vi "NI PXI-4072 DMM Main Page.vi"(8 "error in (no error)":errorcluster, 11 "Node Ptr":T4 format="%.0x") -> (0 "error out":errorcluster)   [LabVIEW 2015, in "NI PXI-4072 DMM Custom Device.lvlib"]
uses:
  NI PXI-4072 DMM Custom Device.lvlib
  <vilib>/NI Veristand/Custom Device API/Custom Device Item Ref.ctl
  4072_CD_DMM Function.ctl
  <vilib>/NI Veristand/Custom Device API/Custom Device Channel.ctl
  <vilib>/NI Veristand/Custom Device API/Custom Device Channel Type.ctl
  4072_Global.vi
  <vilib>/NI Veristand/Custom Device API/Get Item Property (String).vi
  <vilib>/NI Veristand/Custom Device API/Get Item Property (U16).vi
  <vilib>/NI Veristand/Custom Device API/Get Item Property (I32).vi
  <vilib>/NI Veristand/Custom Device API/Set Item Property (U16).vi
  <vilib>/NI Veristand/Custom Device API/Set Item Property (Double).vi
  <vilib>/NI Veristand/Custom Device API/Set Item Property (String).vi
  <vilib>/NI Veristand/Custom Device API/Custom Device API.lvlib
panel:
  in  "Resolution in Digits":T1(ring)=enum."5 1/2"
  in  "Voltage Range":enum16{".1", "1", "10", "100", "300"}(ring)
  in  "Capacitance Range":T2(ring)
  in  "Resistance Range":enum16{"100", "1K", "10K", "1M", "10M", "100M"}(ring)
  in  "Processor":i32=-2 min=-2 max=64 step=1
  in  "Decimation":u16=1
  in  "Measurement Type":T3
  in  "Name of Device in MAX":string
  in  "Header":cluster{"Section Name":string}={"Section Name"="PXI-4072  Settings"}
  in  "Description":string
  in  "Custom Device Name":string
  in  "Delete":bool
  # "(-2 is Automatic)"
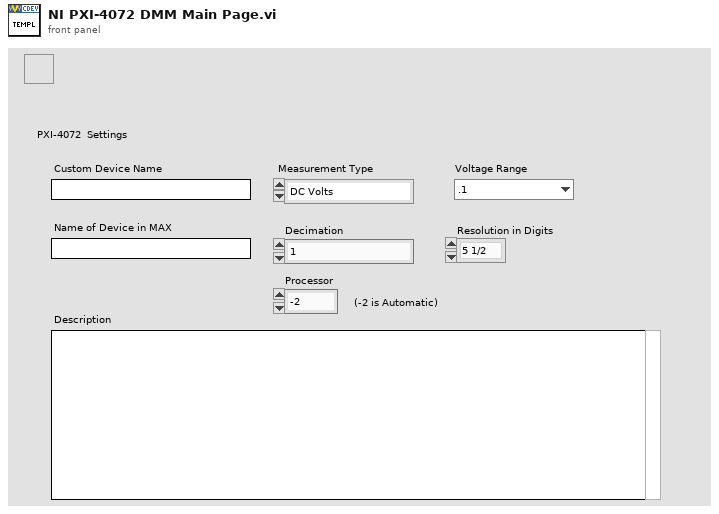
[diagram p1: front panel]
types:
  T1 = enum16{"3 1/2", "4 1/2", "5 1/2", "6 1/2", "7 1/7"}
  T2 = enum16{"300 pF", "1 nF", "10 nF", "100 nF", "1 uF", "10 uF", "100 uF", "1000 uF", "10000 uF"}
  T3 = typedef "NI PXI-4072 DMM Custom Device.lvlib/4072_CD_DMM Function.ctl" = enum16{"DC Volts", "2-wire Resistance", "4-wire Resistance", "Capacitance"}
  T4 = typedef "Custom Device API.lvlib/Custom Device Item Ref.ctl" = u64
  T5 = typedef "Custom Device API.lvlib/Custom Device Channel.ctl" = cluster{"Type":T6, "Units":string, "Default Value":dbl, "Faultable":bool, "Scalable":bool}
  T6 = typedef "Custom Device API.lvlib/Custom Device Channel Type.ctl" = enum16{"Input", "Output"}
  T7 = typedef "Custom Device API.lvlib/Custom Device Item Info.ctl" = cluster{"Name":string, "Is Channel":bool, "GUID":string, "Is Waveform":bool}
  T8 = typedef "Custom Device API.lvlib/Custom Device Commands.ctl" = enum16{"Default", "Item renamed", "Shutdown", "Dynamic button pressed"}
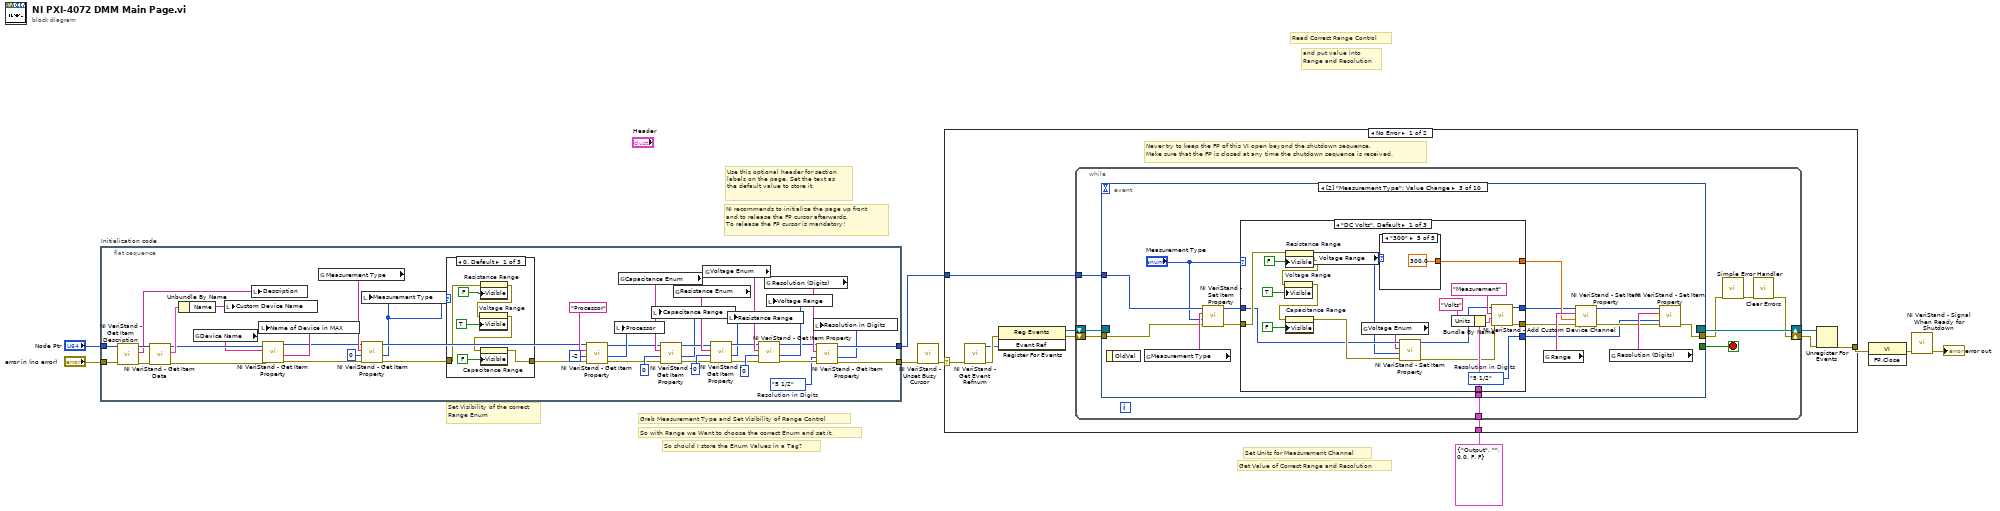
[diagram p0: block diagram]
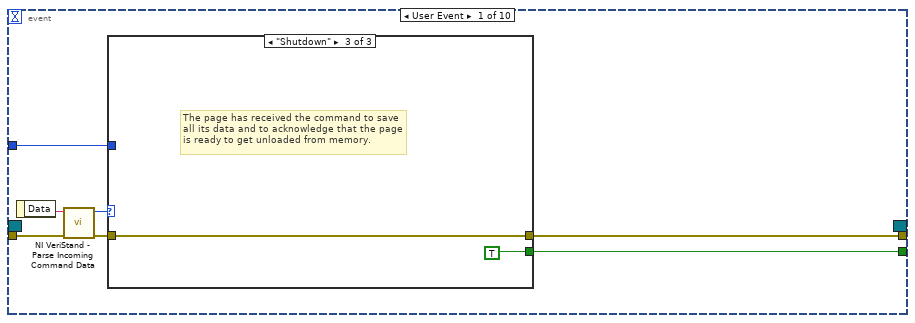
[diagram p2: hidden frame]
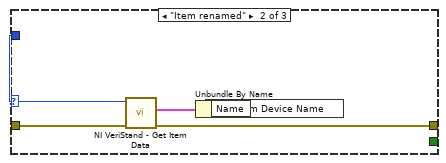
[diagram p4: hidden frame]
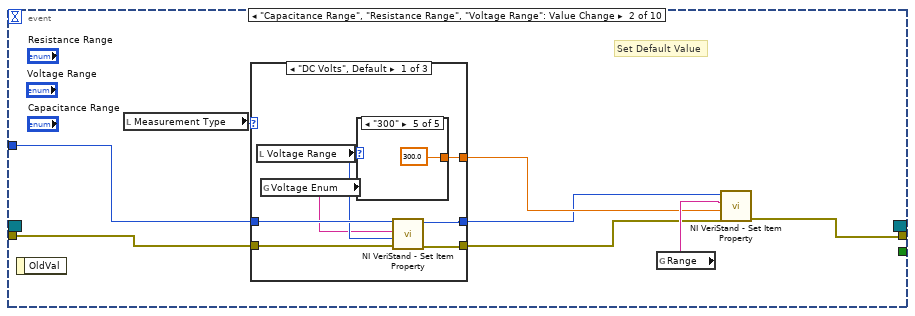
[diagram p5: hidden frame]
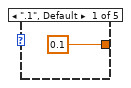
[diagram p6: hidden frame]
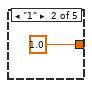
[diagram p7: hidden frame]
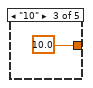
[diagram p8: hidden frame]
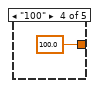
[diagram p9: hidden frame]
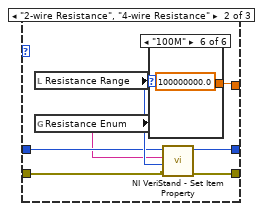
[diagram p10: hidden frame]
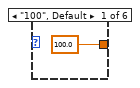
[diagram p11: hidden frame]
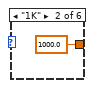
[diagram p12: hidden frame]
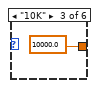
[diagram p13: hidden frame]
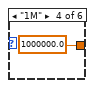
[diagram p14: hidden frame]
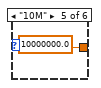
[diagram p15: hidden frame]
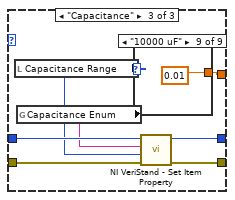
[diagram p16: hidden frame]
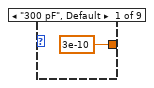
[diagram p17: hidden frame]
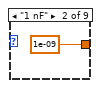
[diagram p18: hidden frame]
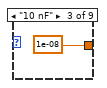
[diagram p19: hidden frame]
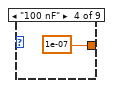
[diagram p20: hidden frame]
diagram:
  # "Set Units for Measurement Channel"
  # "Set Visibility of the correct\nRange Enum"
  # "Get Value of Correct Range and Resolution"
  # "So should I store the Enum Values in a Tag?"
  # "So with Range we Want to choose the correct Enum and set it."
  # "Grab Measurement Type and Set Visibility of Range Control"
  # "and put value into\nRange and Resolution"
  # "Read Correct Range Control"
  # "Use this optional header for section labels on the page. Set the text as the default value to store it."
  # "NI recommends to initialize the page up front\nand to release the FP cursor afterwards.\nTo release the FP cursor is mandatory!"
  n1 = flat-sequence "Initialization code" {
    tunnel: "error in (no error)" -> [w47]
    tunnel: "Node Ptr" -> [w48]
    tunnel: [w34] -> w5
    tunnel: [w35] -> w2
    frame #0 {
      w10 = T1."5 1/2"  # Resolution in Digits
      n2 = call <vilib>:"NI VeriStand - Get Item Description.vi"("error in (no error)"=w47, "Item Ref in"=w48) -> ("error out"=w51:errorcluster, "Description"=w52:string, "Item Ref out"=w53:T4)  [unwired: 7 out]
      n3 = call <vilib>:"NI VeriStand - Get Item Data.vi"("error in (no error)"=w51, "Item Ref in"=w53) -> ("error out"=w46:errorcluster, "Item Info"=w50:T7, "Item Ref out"=w45:T4)  [unwired: 7 out]
      n4 = Unbundle By Name(w50) -> ("Name"=w49:string)
      n5 = global read "4072_Global.vi" "Device Name"() -> (w44:string)
      n6 = local write "Custom Device Name"(w49) -> ()
      n7 = local write "Description"(w52) -> ()
      n8 = call-poly <vilib>:"NI VeriStand - Get Item Property.vi"("error in (no error)"=w46, "Property Name"=w44, "Item Ref in"=w45) -> ("error out"=w41:errorcluster, "Value"=w43:string, "Item Ref out"=w40:T4)  [unwired: 5 in, 1 out]
      n9 = local write "Name of Device in MAX"(w43) -> ()
      n10 = global read "4072_Global.vi" "Measurement Type"() -> (w42:string)
      n11 = call-poly <vilib>:"NI VeriStand - Get Item Property.vi"("error in (no error)"=w41, "Default Value"=u16 0, "Property Name"=w42, "Item Ref in"=w40) -> ("error out"=w13:errorcluster, "Value"=w14:u16, "Item Ref out"=w38:T4)  [unwired: 4 in, 1 out]
      n12 = local write "Measurement Type"(w14) -> ()
      n13 = case shown="0, Default" w14 {
        tunnel: w13 -> [w55 w61 w69]
        tunnel: [w54 w62 w68] -> w12
        frame 0, Default {
          n14 = property on="Resistance Range" class="Enum (strict)"(error in=w55, "Visible"=FALSE) -> (error out=w57:errorcluster)  [unwired: 1 in, 1 out]
          n15 = property on="Voltage Range" class="Enum (strict)"(error in=w57, "Visible"=TRUE) -> (error out=w56:errorcluster)  [unwired: 1 in, 1 out]
          n16 = property on="Capacitance Range" class="Enum (strict)"(error in=w56, "Visible"=FALSE) -> (error out=w54:errorcluster)  [unwired: 1 in, 1 out]
        }
        frame 1, 2 {
          n17 = property on="Resistance Range" class="Enum (strict)"(error in=w61, "Visible"=TRUE) -> (error out=w64:errorcluster)  [unwired: 1 in, 1 out]
          n18 = property on="Voltage Range" class="Enum (strict)"(error in=w64, "Visible"=FALSE) -> (error out=w63:errorcluster)  [unwired: 1 in, 1 out]
          n19 = property on="Capacitance Range" class="Enum (strict)"(error in=w63, "Visible"=FALSE) -> (error out=w62:errorcluster)  [unwired: 1 in, 1 out]
        }
        frame 3 {
          n20 = property on="Resistance Range" class="Enum (strict)"(error in=w69, "Visible"=FALSE) -> (error out=w71:errorcluster)  [unwired: 1 in, 1 out]
          n21 = property on="Voltage Range" class="Enum (strict)"(error in=w71, "Visible"=FALSE) -> (error out=w70:errorcluster)  [unwired: 1 in, 1 out]
          n22 = property on="Capacitance Range" class="Enum (strict)"(error in=w70, "Visible"=TRUE) -> (error out=w68:errorcluster)  [unwired: 1 in, 1 out]
        }
      }
      n23 = call-poly <vilib>:"NI VeriStand - Get Item Property.vi"("error in (no error)"=w12, "Default Value"=-2, "Property Name"="Processor", "Item Ref in"=w38) -> ("error out"=w24:errorcluster, "Value"=w37:i32, "Item Ref out"=w27:T4)  [unwired: 4 in, 1 out]
      n24 = local write "Processor"(w37) -> ()
      n25 = global read "4072_Global.vi" "Capacitance Enum"() -> (w33:string)
      n26 = call-poly <vilib>:"NI VeriStand - Get Item Property.vi"("error in (no error)"=w24, "Default Value"=0, "Property Name"=w33, "Item Ref in"=w27) -> ("error out"=w23:errorcluster, "Value"=w19:u16, "Item Ref out"=w26:T4)  [unwired: 4 in, 1 out]
      n27 = local write "Capacitance Range"(w19) -> ()
      n28 = global read "4072_Global.vi" "Resistance Enum"() -> (w32:string)
      n29 = global read "4072_Global.vi" "Voltage Enum"() -> (w31:string)
      n30 = call-poly <vilib>:"NI VeriStand - Get Item Property.vi"("error in (no error)"=w23, "Default Value"=0, "Property Name"=w32, "Item Ref in"=w26) -> ("error out"=w22:errorcluster, "Value"=w18:u16, "Item Ref out"=w25:T4)  [unwired: 4 in, 1 out]
      n31 = local write "Resistance Range"(w18) -> ()
      n32 = call-poly <vilib>:"NI VeriStand - Get Item Property.vi"("error in (no error)"=w22, "Default Value"=0, "Property Name"=w31, "Item Ref in"=w25) -> ("error out"=w21:errorcluster, "Value"=w20:u16, "Item Ref out"=w17:T4)  [unwired: 4 in, 1 out]
      n33 = global read "4072_Global.vi" "Resolution (Digits)"() -> (w36:string)
      n34 = local write "Voltage Range"(w20) -> ()
      n35 = call-poly <vilib>:"NI VeriStand - Get Item Property.vi"("error in (no error)"=w21, "Default Value"=w10, "Property Name"=w36, "Item Ref in"=w17) -> ("error out"=w34:errorcluster, "Value"=w11:u16, "Item Ref out"=w35:T4)  [unwired: 4 in, 1 out]
      n36 = local write "Resolution in Digits"(w11) -> ()
    }
  }
  n37 = call <vilib>:"NI VeriStand - Unset Busy Cursor.vi"("error in (no error)"=w5) -> ("error out"=w4:errorcluster)  [unwired: 10 out]
  n38 = case shown="No Error" w4 {
    selector: w4 -> [w76 w286]
    tunnel: [w81 w284] -> w9
    tunnel: w2 -> [w77 _]
    tunnel: T5 {"Type"=enum."Output", "Units"="", "Default Value"=0.0, "Faultable"=FALSE, "Scalable"=FALSE} ("Channel") -> [w75 _]
    frame No Error {
      # "Never try to keep the FP of this VI open beyond the shutdown sequence.\nMake sure that the FP is closed at any time the shutdown sequence is received."
      n39 = call <vilib>:"NI VeriStand - Get Event Refnum.vi"("error in (no error)"=w76) -> ("error out"=w84:errorcluster, "Event Ref"=w80:refnum<user-event>)  [unwired: 9 out]
      n40 = register-events(error in=w84, w80) -> (reference out=w78:refnum<event-registration>, error out=w79:errorcluster)  [unwired: 1 in]
      n41 = while {
        tunnel: w77 -> [w89]
        shift-right: [w86] -> w82
        shift-left: w79 -> [w92]
        shift-right: [w93] -> w83
        shift-left: w78 -> [w91]
        tunnel: w75 -> [w85]
        stop <- w90 stop-if-true
        n42 = event shown="[2] \"Measurement Type\": Value Change" {
          selector: w91 -> [_ _ _ _ _ _ _ _ _ _]
          dyn-events: [_ _ _ _ _ _ _ _ _ _] -> w93
          timeout: _ -> [_ _ _ _ _ _ _ _ _ _]
          tunnel: w92 -> [w100 w111 w170 w256 w260 w265 w272 w276 w279 w283]
          tunnel: [w96 _ _ _ _ _ _ _ _ _] -> w90
          tunnel: [w95 w114 w164 w255 w259 w264 w268 w275 w278 w282] -> w88
          tunnel: w89 -> [w94 w112 w171 w257 w262 w266 w271 w274 w280 w281]
          tunnel: w85 -> [_ _ w158 _ _ _ _ _ _ _]
          event User Event {
            n43 = event-data() -> ("Data"=w99:string)  [unwired: 1 out]
            n44 = call <vilib>:"NI VeriStand - Parse Incoming Command Data.vi"("error in (no error)"=w100, "Incoming data"=w99) -> ("error out"=w98:errorcluster, "Action"=w97:T8)  [unwired: 8 out]
            n45 = case shown="\"Shutdown\"" w97 {
              tunnel: w98 -> [w101 w106 w107]
              tunnel: [_ _ TRUE] -> w96
              tunnel: [w101 w103 w107] -> w95
              tunnel: w94 -> [_ w105 _]
              frame "Default", Default {
              }
              frame "Item renamed" {
                n46 = call <vilib>:"NI VeriStand - Get Item Data.vi"("error in (no error)"=w106, "Item Ref in"=w105) -> ("error out"=w103:errorcluster, "Item Info"=w104:T7)  [unwired: 8 out]
                n47 = Unbundle By Name(w104) -> ("Name"=w102:string)
                n48 = local write "Custom Device Name"(w102) -> ()
              }
              frame "Shutdown" {
                # "The page has received the command to save all its data and to acknowledge that the page is ready to get unloaded from memory."
              }
            }
          }
          event "Capacitance Range", "Resistance Range", "Voltage Range": Value Change {
            # "Set Default Value"
            n49 = event-data() -> ()  [unwired: 2 out]
            n50 = local read "Measurement Type"() -> (w116:T3)
            n51 = case shown="\"DC Volts\", Default" w116 {
              tunnel: [w123 w135 w148] -> w113
              tunnel: w112 -> [w119 w133 w147]
              tunnel: w111 -> [w120 w130 w146]
              tunnel: [w121 w131 w145] -> w110
              tunnel: [w122 w132 w144] -> w109
              frame "DC Volts", Default {
                n52 = local read "Voltage Range"() -> (w118:enum16{".1", "1", "10", "100", "300"})
                n53 = global read "4072_Global.vi" "Voltage Enum"() -> (w117:string)
                n54 = case shown="\"300\"" w118 {
                  tunnel: [0.1 1.0 10.0 100.0 300.0] -> w123
                  frame ".1", Default {
                  }
                  frame "1" {
                  }
                  frame "10" {
                  }
                  frame "100" {
                  }
                  frame "300" {
                  }
                }
                n55 = call-poly <vilib>:"NI VeriStand - Set Item Property.vi"("error in (no error)"=w120, "Value"=w118, "Property Name"=w117, "Item Ref in"=w119) -> ("error out"=w121:errorcluster, "Item Ref out"=w122:T4)  [unwired: 5 in, 1 out]
              }
              frame "2-wire Resistance", "4-wire Resistance" {
                n56 = local read "Resistance Range"() -> (w134:enum16{"100", "1K", "10K", "1M", "10M", "100M"})
                n57 = global read "4072_Global.vi" "Resistance Enum"() -> (w129:string)
                n58 = case shown="\"100M\"" w134 {
                  tunnel: [100.0 1000.0 10000.0 1000000.0 10000000.0 100000000.0] -> w135
                  frame "100", Default {
                  }
                  frame "1K" {
                  }
                  frame "10K" {
                  }
                  frame "1M" {
                  }
                  frame "10M" {
                  }
                  frame "100M" {
                  }
                }
                n59 = call-poly <vilib>:"NI VeriStand - Set Item Property.vi"("error in (no error)"=w130, "Value"=w134, "Property Name"=w129, "Item Ref in"=w133) -> ("error out"=w131:errorcluster, "Item Ref out"=w132:T4)  [unwired: 5 in, 1 out]
              }
              frame "Capacitance" {
                n60 = local read "Capacitance Range"() -> (w142:T2)
                n61 = global read "4072_Global.vi" "Capacitance Enum"() -> (w143:string)
                n62 = case shown="\"10000 uF\"" w142 {
                  tunnel: [3e-10 1e-09 1e-08 1e-07 1e-06 1e-05 0.0001 0.001 0.01] -> w148
                  frame "300 pF", Default {
                  }
                  frame "1 nF" {
                  }
                  frame "10 nF" {
                  }
                  frame "100 nF" {
                  }
                  frame "1 uF" {
                  }
                  frame "10 uF" {
                  }
                  frame "100 uF" {
                  }
                  frame "1000 uF" {
                  }
                  frame "10000 uF" {
                  }
                }
                n63 = call-poly <vilib>:"NI VeriStand - Set Item Property.vi"("error in (no error)"=w146, "Value"=w142, "Property Name"=w143, "Item Ref in"=w147) -> ("error out"=w145:errorcluster, "Item Ref out"=w144:T4)  [unwired: 5 in, 1 out]
              }
            }
            n64 = global read "4072_Global.vi" "Range"() -> (w115:string)
            n65 = call-poly <vilib>:"NI VeriStand - Set Item Property.vi"("error in (no error)"=w110, "Value"=w113, "Property Name"=w115, "Item Ref in"=w109) -> ("error out"=w114:errorcluster)  [unwired: 5 in, 2 out]
          }
          event Value Change {
            n66 = event-data() -> ()  [unwired: 2 out]
            n67 = global read "4072_Global.vi" "Measurement Type"() -> (w173:string)
            n68 = call-poly <vilib>:"NI VeriStand - Set Item Property.vi"("error in (no error)"=w170, "Value"="Measurement Type", "Property Name"=w173, "Item Ref in"=w171) -> ("error out"=w172:errorcluster, "Item Ref out"=w160:T4)  [unwired: 5 in, 1 out]
            n69 = case shown="\"DC Volts\", Default" "Measurement Type" {
              tunnel: w172 -> [w190 w215 w241]
              tunnel: [w180 w205 w226] -> w165
              tunnel: [w187 w212 w238] -> w162
              tunnel: [w174 w199 w225] -> w161
              tunnel: w160 -> [w185 w210 w235]
              tunnel: [w181 w206 w227] -> w159
              tunnel: w158 -> [w179 w202 w232]
              frame "DC Volts", Default {
                w174 = T1."5 1/2"  # Resolution in Digits
                n70 = property on="Resistance Range" class="Enum (strict)"(error in=w190, "Visible"=FALSE) -> (error out=w189:errorcluster)  [unwired: 1 in, 1 out]
                n71 = property on="Voltage Range" class="Enum (strict)"(error in=w189, "Visible"=TRUE) -> (error out=w188:errorcluster)  [unwired: 1 in, 1 out]
                n72 = property on="Capacitance Range" class="Enum (strict)"(error in=w188, "Visible"=FALSE) -> (error out=w186:errorcluster)  [unwired: 1 in, 1 out]
                n73 = local read "Voltage Range"() -> (w183:enum16{".1", "1", "10", "100", "300"})
                n74 = global read "4072_Global.vi" "Voltage Enum"() -> (w184:string)
                n75 = case shown="\"300\"" w183 {
                  tunnel: [0.1 1.0 10.0 100.0 300.0] -> w187
                  frame ".1", Default {
                  }
                  frame "1" {
                  }
                  frame "10" {
                  }
                  frame "100" {
                  }
                  frame "300" {
                  }
                }
                n76 = call-poly <vilib>:"NI VeriStand - Set Item Property.vi"("error in (no error)"=w186, "Value"=w183, "Property Name"=w184, "Item Ref in"=w185) -> ("error out"=w176:errorcluster, "Item Ref out"=w175:T4)  [unwired: 5 in, 1 out]
                n77 = Bundle By Name(cluster=w179, "Units"="Volts") -> (w178:T5)
                n78 = call <vilib>:"NI VeriStand - Add Custom Device Channel.vi"("error in (no error)"=w176, "Channel"=w178, "Channel Name"="Measurement", "Parent Ref in"=w175) -> ("error out"=w180:errorcluster, "Parent Ref out"=w181:T4)  [unwired: 4 in, 2 out]
              }
              frame "2-wire Resistance", "4-wire Resistance" {
                n79 = global read "4072_Global.vi" "Resistance Enum"() -> (w208:string)
                n80 = property on="Resistance Range" class="Enum (strict)"(error in=w215, "Visible"=TRUE) -> (error out=w214:errorcluster)  [unwired: 1 in, 1 out]
                n81 = property on="Voltage Range" class="Enum (strict)"(error in=w214, "Visible"=FALSE) -> (error out=w213:errorcluster)  [unwired: 1 in, 1 out]
                n82 = property on="Capacitance Range" class="Enum (strict)"(error in=w213, "Visible"=FALSE) -> (error out=w211:errorcluster)  [unwired: 1 in, 1 out]
                n83 = local read "Resistance Range"() -> (w209:enum16{"100", "1K", "10K", "1M", "10M", "100M"})
                n84 = local read "Resolution in Digits"() -> (w199:T1)
                n85 = case shown="\"1K\"" w209 {
                  tunnel: [100.0 1000.0 10000.0 1000000.0 10000000.0 100000000.0] -> w212
                  frame "100", Default {
                  }
                  frame "1K" {
                  }
                  frame "10K" {
                  }
                  frame "1M" {
                  }
                  frame "10M" {
                  }
                  frame "100M" {
                  }
                }
                n86 = call-poly <vilib>:"NI VeriStand - Set Item Property.vi"("error in (no error)"=w211, "Value"=w209, "Property Name"=w208, "Item Ref in"=w210) -> ("error out"=w204:errorcluster, "Item Ref out"=w203:T4)  [unwired: 5 in, 1 out]
                n87 = Bundle By Name(cluster=w202, "Units"="Ohms") -> (w201:T5)
                n88 = call <vilib>:"NI VeriStand - Add Custom Device Channel.vi"("error in (no error)"=w204, "Channel"=w201, "Channel Name"="Measurement", "Parent Ref in"=w203) -> ("error out"=w205:errorcluster, "Parent Ref out"=w206:T4)  [unwired: 4 in, 2 out]
              }
              frame "Capacitance" {
                w225 = T1."5 1/2"  # Resolution in Digits
                n89 = property on="Resistance Range" class="Enum (strict)"(error in=w241, "Visible"=FALSE) -> (error out=w240:errorcluster)  [unwired: 1 in, 1 out]
                n90 = global read "4072_Global.vi" "Capacitance Enum"() -> (w234:string)
                n91 = property on="Voltage Range" class="Enum (strict)"(error in=w240, "Visible"=FALSE) -> (error out=w239:errorcluster)  [unwired: 1 in, 1 out]
                n92 = local read "Capacitance Range"() -> (w237:T2)
                n93 = property on="Capacitance Range" class="Enum (strict)"(error in=w239, "Visible"=TRUE) -> (error out=w236:errorcluster)  [unwired: 1 in, 1 out]
                n94 = case shown="\"10000 uF\"" w237 {
                  tunnel: [3e-10 1e-09 1e-08 1e-07 1e-06 1e-05 0.0001 0.001 0.01] -> w238
                  frame "300 pF", Default {
                  }
                  frame "1 nF" {
                  }
                  frame "10 nF" {
                  }
                  frame "100 nF" {
                  }
                  frame "1 uF" {
                  }
                  frame "10 uF" {
                  }
                  frame "100 uF" {
                  }
                  frame "1000 uF" {
                  }
                  frame "10000 uF" {
                  }
                }
                n95 = call-poly <vilib>:"NI VeriStand - Set Item Property.vi"("error in (no error)"=w236, "Value"=w237, "Property Name"=w234, "Item Ref in"=w235) -> ("error out"=w229:errorcluster, "Item Ref out"=w228:T4)  [unwired: 5 in, 1 out]
                n96 = Bundle By Name(cluster=w232, "Units"="Farads") -> (w231:T5)
                n97 = call <vilib>:"NI VeriStand - Add Custom Device Channel.vi"("error in (no error)"=w229, "Channel"=w231, "Channel Name"="Measurement", "Parent Ref in"=w228) -> ("error out"=w226:errorcluster, "Parent Ref out"=w227:T4)  [unwired: 4 in, 2 out]
              }
            }
            n98 = global read "4072_Global.vi" "Range"() -> (w168:string)
            n99 = call-poly <vilib>:"NI VeriStand - Set Item Property.vi"("error in (no error)"=w165, "Value"=w162, "Property Name"=w168, "Item Ref in"=w159) -> ("error out"=w167:errorcluster, "Item Ref out"=w166:T4)  [unwired: 5 in, 1 out]
            n100 = global read "4072_Global.vi" "Resolution (Digits)"() -> (w169:string)
            n101 = call-poly <vilib>:"NI VeriStand - Set Item Property.vi"("error in (no error)"=w167, "Value"=w161, "Property Name"=w169, "Item Ref in"=w166) -> ("error out"=w164:errorcluster)  [unwired: 5 in, 2 out]
          }
          event "Resolution in Digits": Value Change {
            n102 = event-data() -> ()  [unwired: 4 out]
            n103 = global read "4072_Global.vi" "Resolution (Digits)"() -> (w258:string)
            n104 = call-poly <vilib>:"NI VeriStand - Set Item Property.vi"("error in (no error)"=w256, "Value"="Resolution in Digits", "Property Name"=w258, "Item Ref in"=w257) -> ("error out"=w255:errorcluster)  [unwired: 5 in, 2 out]
          }
          event "Decimation": Value Change {
            n105 = event-data() -> ()  [unwired: 2 out]
            n106 = call <vilib>:"NI VeriStand - Set Custom Device Decimation.vi"("error in (no error)"=w260, "Decimation"="Decimation", "Device Ref in"=w262) -> ("error out"=w259:errorcluster)  [unwired: 7 in, 1 out]
          }
          event "Processor": Value Change {
            n107 = event-data() -> ()  [unwired: 2 out]
            n108 = call-poly <vilib>:"NI VeriStand - Get Item Property.vi"("error in (no error)"=w265, "Default Value"="Processor", "Property Name"="Processor", "Item Ref in"=w266) -> ("error out"=w264:errorcluster)  [unwired: 4 in, 3 out]
          }
          event "Name of Device in MAX": Value Change {
            n109 = event-data() -> ()  [unwired: 2 out]
            n110 = global read "4072_Global.vi" "Device Name"() -> (w270:string)
            n111 = call-poly <vilib>:"NI VeriStand - Set Item Property.vi"("error in (no error)"=w272, "Value"="Name of Device in MAX", "Property Name"=w270, "Item Ref in"=w271) -> ("error out"=w268:errorcluster)  [unwired: 5 in, 2 out]
          }
          event "Custom Device Name": Value Change {
            n112 = event-data() -> ()  [unwired: 2 out]
            n113 = call <vilib>:"NI VeriStand - Rename Custom Device Item.vi"("error in (no error)"=w276, "New Name"="Custom Device Name", "Item Ref in"=w274) -> ("error out"=w275:errorcluster)  [unwired: 1 in, 7 out]
          }
          event "Description": Value Change {
            n114 = event-data() -> ()  [unwired: 2 out]
            n115 = call <vilib>:"NI VeriStand - Set Item Description.vi"("error in (no error)"=w279, "Description"="Description", "Item Ref in"=w280) -> ("error out"=w278:errorcluster)  [unwired: 8 out]
          }
          event "Delete": Value Change {
            # "If you call the Remove Item, it is highly recommended\nthat the Node Ptr that is connected as input is the Node Ptr of\nthe currenct page. The Remove Item sequence will automatically\nselect the next item in the tree.\n\nRemove Item will delete the selected item and any child items."
            n116 = event-data() -> ()  [unwired: 2 out]
            n117 = call <vilib>:"NI VeriStand - Remove Custom Device Item.vi"("error in (no error)"=w283, "Item Ref in"=w281) -> ("error out"=w282:errorcluster)  [unwired: 1 in, 8 out]
          }
        }
        n118 = call <vilib>:"Simple Error Handler.vi"("error in (no error)"=w88) -> ("error out"=w87:errorcluster)  [unwired: 1 in, 7 out]
        n119 = call <vilib>:"Clear Errors.vi"("error in (no error)"=w87) -> ("error out"=w86:errorcluster)  [unwired: 1 in, 5 out]
      }
      n120 = Unregister For Events(event registration refnum=w83, error in=w82) -> (error out=w81:errorcluster)
    }
    frame Error {
      n121 = call <vilib>:"Simple Error Handler.vi"("error in (no error)"=w286) -> ("error out"=w285:errorcluster)  [unwired: 1 in, 7 out]
      n122 = call <vilib>:"Clear Errors.vi"("error in (no error)"=w285) -> ("error out"=w284:errorcluster)  [unwired: 1 in, 5 out]
    }
  }
  n123 = invoke class="VI" method="FP.Close"(error in=w9) -> (error out=w8:errorcluster)  [unwired: 2 in, 2 out]
  n124 = call <vilib>:"NI VeriStand - Signal When Ready for Shutdown.vi"("error in (no error)"=w8) -> ("error out"=→"error out":errorcluster)  [unwired: 10 out]
